vi "Dictionary.Remove Empty.vi"(8 "error in (no error)":errorcluster, 10 "Data (Dictionary)":T1[](array[typedef])) -> (0 "error out":errorcluster, 1 "max Array Size":i32, 2 "Data (Dictionary)":T1[](array[typedef]))   [LabVIEW 2019, in "Conversion.lvclass"]
uses:
  Conversion.lvclass
  <vilib>/Utility/Data Type/NI_Data Type.lvlib
  Data/Typedefs/Dictionary--cluster.ctl
  Data/Data.lvclass
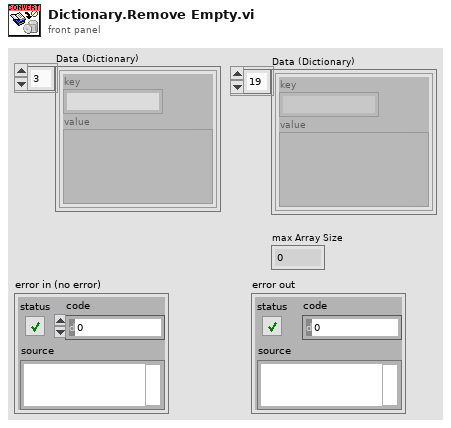
[diagram p1: front panel]
types:
  T1 = typedef "Data.lvclass/Dictionary--cluster.ctl" = cluster{"key":string, "value":variant}
  T2 = typedef "NI_Data Type.lvlib/Data Type.ctl" = enum8{"Invalid Type", "Void", "I8", "I16", "I32", "I64", "U8", "U16", "U32", "U64", "Single Float", "Double Float", "Extended Float", "Single Complex", "Double Complex", "Extended Complex", "Enum U8", "Enum U16", "Enum U32", "Enum U64", "Single Float With Unit", "Double Float With Unit", "Extended Float With Unit", "Single Complex with Unit", "Double Complex with Unit", "Extended Complex with Unit", "Boolean", "String", "Path", "Picture", "Tag", "Array", "Cluster", "Variant", "LV Variant", "Waveform", "Timestamp", "Digital Waveform", "Digital Data", "ExpressData", "Refnum", "External Data", "VI", "Poly VI", "LabVIEW Class Instance", "Fixed Point", "Set Collection", "Map Collection"}
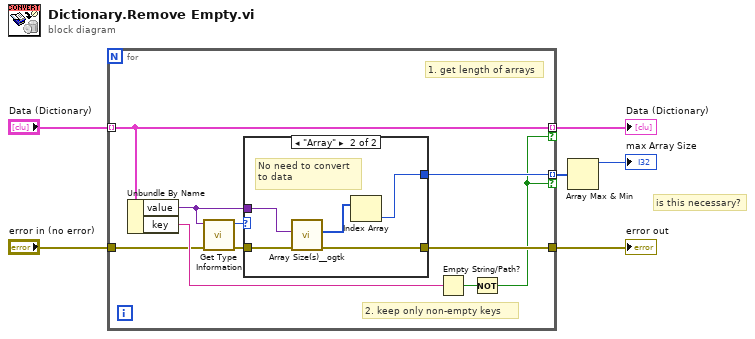
[diagram p0: block diagram]
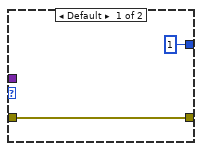
[diagram p2: hidden frame]
diagram:
  # "is this necessary?"
  n1 = for {
    tunnel: "Data (Dictionary)" -> [w8] mode=indexing
    tunnel: [w15] -> w6 mode=indexing if=w7
    tunnel: [w8] -> w5 mode=indexing if=w7
    tunnel: [w14] -> w1
    tunnel: "error in (no error)" -> [w10]
    # "2. keep only non-empty keys"
    # "1. get length of arrays"
    n2 = Unbundle By Name(w8) -> ("value"=w12:variant, "key"=w13:string)
    n3 = call <vilib>:"Get Type Information.vi"("error in (no error)"=w10, "variant"=w12) -> ("error out"=w9:errorcluster, "type"=w11:T2)  [unwired: 5 in, 3 out]
    n4 = case shown="\"Array\"" w11 {
      tunnel: [1 w19] -> w15
      tunnel: w9 -> [w17 w22]
      tunnel: [w17 w20] -> w14
      tunnel: w12 -> [_ w21]
      frame Default {
      }
      frame "Array" {
        # "No need to convert\nto data"
        n5 = call "Array Size(s)__ogtk.vi"("error in (no error)"=w22, "Array"=w21) -> ("error out"=w20:errorcluster, "Size(s)"=w23:u32[])  [unwired: 7 in, 1 out]
        n6 = Index Array(array=w23) -> (element=w19:u32)  [unwired: 1 in]
      }
    }
    n7 = Empty String/Path?(string/path=w13) -> (empty?=w16:bool)
    n8 = Not(x=w16) -> (.not. x?=w7:bool)
  }
  "error out" <- w1
  "Data (Dictionary)" <- w5
  n9 = Array Max & Min(array=w6) -> (max value=→"max Array Size":u32)  [unwired: 3 out]
